vi "Cost.vi"(0 "reference in":refnum<class "Espresso.lvclass">, 5 "error in (no error)":errorcluster) -> (14 "reference out":refnum<class "Espresso.lvclass">, 16 "Cost($)":dbl, 19 "error out":errorcluster)   [LabVIEW 2020, in "Espresso.lvclass"]
uses:
  Espresso.lvclass
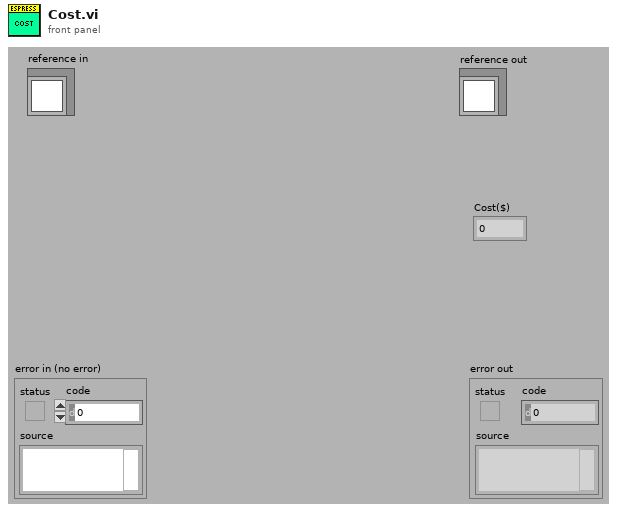
[diagram p1: front panel]
types:
  T1 = typedef "Espresso.lvclass/ObjectAttributes.ctl" = cluster{"None":bool}
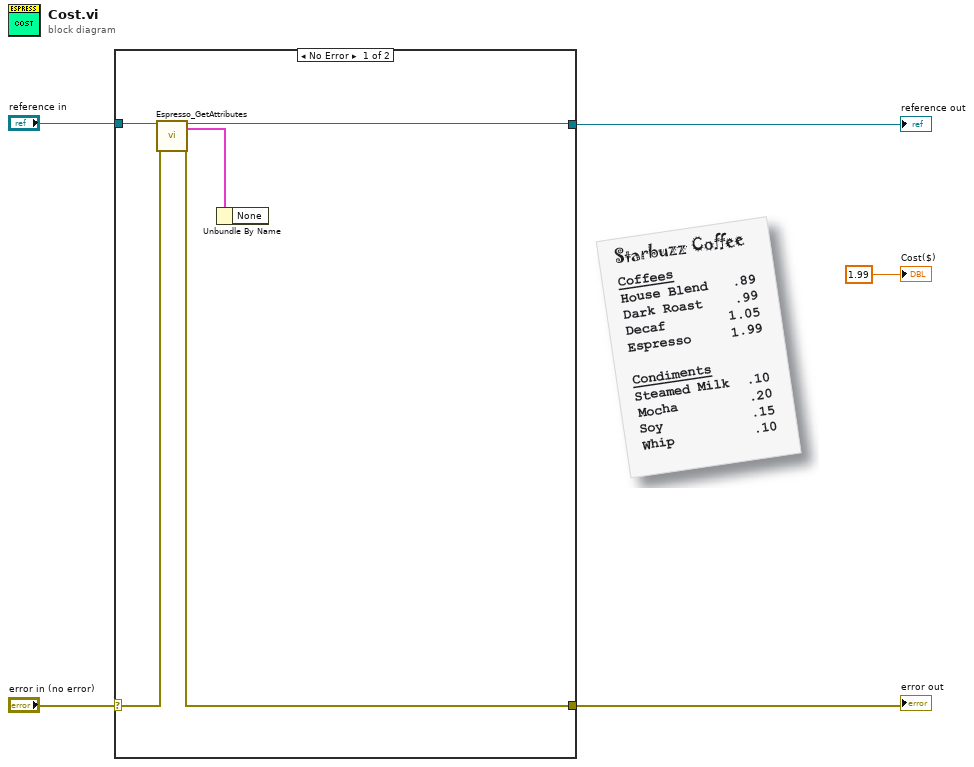
[diagram p0: block diagram]
diagram:
  n1 = case shown="No Error" "error in (no error)" {
    selector: "error in (no error)" -> [w9 w12]
    tunnel: [w6 w12] -> w4
    tunnel: [w7 w11] -> w2
    tunnel: "reference in" -> [w10 w11]
    frame No Error {
      n2 = call "Espresso_GetAttributes.vi"("reference in"=w10, "error in (no error)"=w9) -> ("reference out"=w7:refnum<class "Espresso.lvclass">, "Data"=w8:T1, "error out"=w6:errorcluster)  [unwired: 14 in, 1 out]
      n3 = Unbundle By Name(w8) -> ()  [unwired: 1 out]
    }
    frame Error {
    }
  }
  "error out" <- w4
  "reference out" <- w2
  "Cost($)" <- 1.99 ("Cost($)")
